vi "INI_BLE.vi"(3 "MCListbox Ref":refnum<vi>, 8 "MListBox Row":u16=2 max=8, 10 "Device INI Config File Path":path=path "D:/LABVIEW/SEQUENSER_SNA/Ver_12/INI/DeviceConfig.ini") -> (0 "error out":errorcluster, 1 "ComPort":refnum<visa-resource-name>, 2 "Dev OK":bool)   [LabVIEW 2018]
uses:
  <vilib>/Utility/miscctls.llb/LVRowAndColumnTypeDef.ctl
  <vilib>/Utility/config.llb/Read Key (String).vi
  <vilib>/Utility/config.llb/NI_LVConfig.lvlib
panel:
  out "Dev Description":string=" (???)"
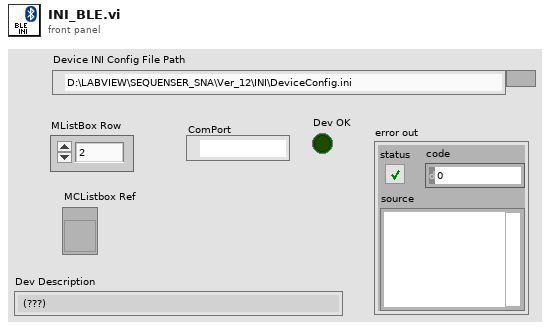
[diagram p1: front panel]
types:
  T1 = typedef "LVRowAndColumnTypeDef.ctl" = cluster{"Row":i32, "Column":i32}
  T2 = typedef "NI_LVConfig.lvlib/Config Data RefNum.ctl" = refnum<k1>
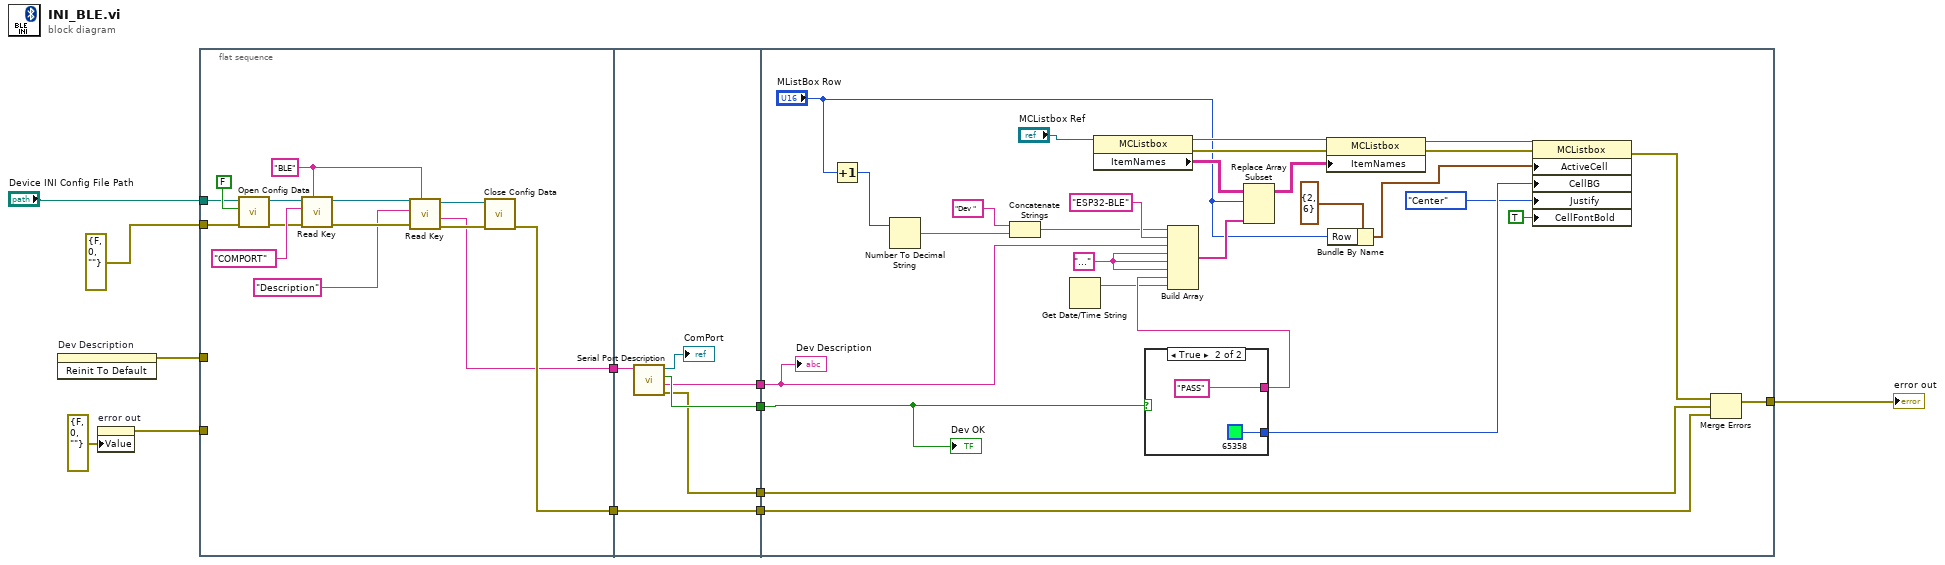
[diagram p0: block diagram]
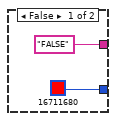
[diagram p2: hidden frame]
diagram:
  n1 = invoke on="Dev Description" class="Str" method="Reinit To Default"() -> (error out=w1:errorcluster)  [unwired: 3 in, 2 out]
  n2 = property on="error out" class="Clust (strict)"("Value"=errorcluster {"status"=FALSE, "code"=0, "source"=""} ("error out")) -> (error out=w9:errorcluster)  [unwired: 2 in, 1 out]
  n3 = flat-sequence {
    tunnel: "Device INI Config File Path" -> [w22]
    tunnel: [w21] -> w12
    tunnel: w9 -> [_]
    tunnel: errorcluster {"status"=FALSE, "code"=0, "source"=""} ("error constant") -> [w20]
    tunnel: [w14] -> w5
    tunnel: w1 -> [_]
    tunnel: w12 -> [w29]
    tunnel: [w31] -> w10
    tunnel: w5 -> [w28]
    tunnel: [w32] -> w4
    tunnel: [w27] -> w3
    tunnel: [w29] -> w2
    tunnel: [w36] -> w7
    tunnel: w10 -> [w34]
    tunnel: w4 -> [w39]
    tunnel: w3 -> [w37]
    tunnel: w2 -> [w33]
    frame #0 {
      w15 = "BLE" ("section")
      n4 = call <vilib>:"Open Config Data.vi"("error in (no error)"=w20, "create file if necessary (T)"=FALSE, "configuration file path"=w22) -> ("error out"=w25:errorcluster, "refnum"=w24:T2)  [unwired: 6 in, 1 out]
      n5 = call-poly <vilib>:"Read Key.vi"("section"=w15, "error in (no error)"=w25, "key"="COMPORT", "refnum"=w24) -> ("error out"=w17:errorcluster, "refnum out"=w19:T2)  [unwired: 4 in, 2 out]
      n6 = call-poly <vilib>:"Read Key.vi"("section"=w15, "error in (no error)"=w17, "key"="Description", "refnum"=w19) -> ("error out"=w16:errorcluster, "value"=w14:string, "refnum out"=w18:T2)  [unwired: 4 in, 1 out]
      n7 = call <vilib>:"Close Config Data.vi"("error in (no error)"=w16, "refnum"=w18) -> ("error out"=w21:errorcluster)  [unwired: 8 in, 1 out]
    }
    frame #1 {
      n8 = call "Serial Port Description.vi"("Dev Description"=w28) -> ("error out"=w31:errorcluster, "Dev Description"=w27:string, "OK?"=w32:bool, "VISA resource name"=→"ComPort":refnum<visa-resource-name>)  [unwired: 7 in]
    }
    frame #2 {
      w38 = "..."
      n9 = Increment(x="MListBox Row") -> (x+1=w41:u16)
      n10 = Number To Decimal String(number=w41) -> (decimal integer string=w58:string)  [unwired: 1 in]
      n11 = Concatenate Strings("Dev ", w58) -> (w59:string)
      n12 = Get Date/Time String() -> (date string=w51:string)  [unwired: 3 in, 1 out]
      n13 = property class="MCListbox"(reference="MCListbox Ref") -> (reference out=w49:refnum<vi>, error out=w48:errorcluster, "ItemNames"=w47:string[][])  [unwired: 1 in]
      n14 = case shown="True" w39 {
        tunnel: [u32 16711680 u32 65358] -> w54
        tunnel: ["FALSE" ("element") "PASS" ("element")] -> w55
        frame False {
        }
        frame True {
        }
      }
      n15 = Build Array(w59, "ESP32-BLE", w37, w38, w38, w38, w55, w51) -> (w45:string[])
      n16 = Replace Array Subset(array=w47, new element=w45, index (row)="MListBox Row") -> (w46:string[][])  [unwired: 1 in]
      n17 = property class="MCListbox"(reference=w49, error in=w48, "ItemNames"=w46) -> (reference out=w44:refnum<vi>, error out=w43:errorcluster)
      n18 = Bundle By Name(cluster=T1 {"Row"=2, "Column"=6} ("Active Cell:Active Cell"), "Row"="MListBox Row") -> (w53:T1)
      n19 = property class="MCListbox"(reference=w44, error in=w43, "ActiveCell"=w53, "CellBG"=w54, "Justify"=enum16{"Left", "Center", "Right"}."Center" ("Active Cell:Cell Justification"), "CellFontBold"=TRUE ("Active Cell:Cell Font:Bold")) -> (error out=w35:errorcluster)  [unwired: 1 out]
      n20 = Merge Errors(w35, w34, w33) -> (w36:errorcluster)
      "Dev OK" <- w39
      "Dev Description" <- w37
    }
  }
  "error out" <- w7
